vi "AGE_Machine_Interface_v6.vi"() -> ()   [LabVIEW 2016]
uses:
  <vilib>/Analysis/3filter.llb/Filter Passband Type.ctl
  <vilib>/instr/_visa.llb/VISA Configure Serial Port (Instr).vi
  <vilib>/ptbypt/NI_PtbyPt.lvlib
  <vilib>/Analysis/NI_AALBase.lvlib
panel:
  out "input variable":dbl
  out "output variable":dbl
  out "Winds Completed":dbl
  out "Total Number of Winds":dbl
  out "sh_r-new":dbl
  out "winds\ncompleted":i32
  out "Roboteq":refnum<visa-resource-name>
  out "Interface Information:Interface Description 2":string
  out "General Settings:Resource Name 2":string
  out "General Settings:Resource Name":string
  out "Interface Information:Interface Description":string
  out "Uno":refnum<visa-resource-name>
  out "List of card in the Computer 2":string[](array[string])
  out "List of card in the Computer":string[](array[string])
  in  "Start Button":bool
  out "READY":bool
  out "INITIALIZING":bool
  out "NOT READY":bool
  in  "Glue Cart":bool
  in  "Fiber Roll":bool
  in  "Acrylic Tube":bool
  out "sh_r":dbl format="%#_5g"
  out "AGE Fiber Outer Diameter [mm]":dbl format="%#_3g"
  out "AGE Length of Roll Wound [m]":dbl format="%#_3g"
  out "AGE Number of Fiber Layers":dbl format="%#_3g"
  out "AGE Length of Roll Wound [ft]":dbl format="%#_3g"
  out "AGE Fiber Outer Diameter [in]":dbl format="%#_3g"
  in  "AGE Fiber \nSurface Area [m^2]":dbl=1.0
  in  "AGE Effective Width [mm]":dbl=50.0
  in  "AGE Initial \nDiameter [in]":dbl=1.0
  out "Quantity Glue":dbl=23.78296263980416 format="%#_2g"
  in  "Motors Stop":bool
  in  "?":bool
  out "error out 2":errorcluster
  out "Ready 2":bool
  out "Ready":bool
  in  "?":bool
  out "error out":errorcluster
  in  "Calculate\nCalculate Button":bool
  in  "Reset Button":bool
  # "AGE Winding Machine Interface"
  # "Serial Port\nStatus"
  # "Setup Operation"
  # "Stepper\nMotor"
  # "Glue Quantity Per Cartridge"
  # "[mL]"
  # "Glue &Wind Motor"
  # "ENTER THE VALUES AND THEN PRESS CALCULATE"
  # "Calculation Outputs"
  # "CHECK THE BOXES IF CRITERIA IS MET BEFORE START"
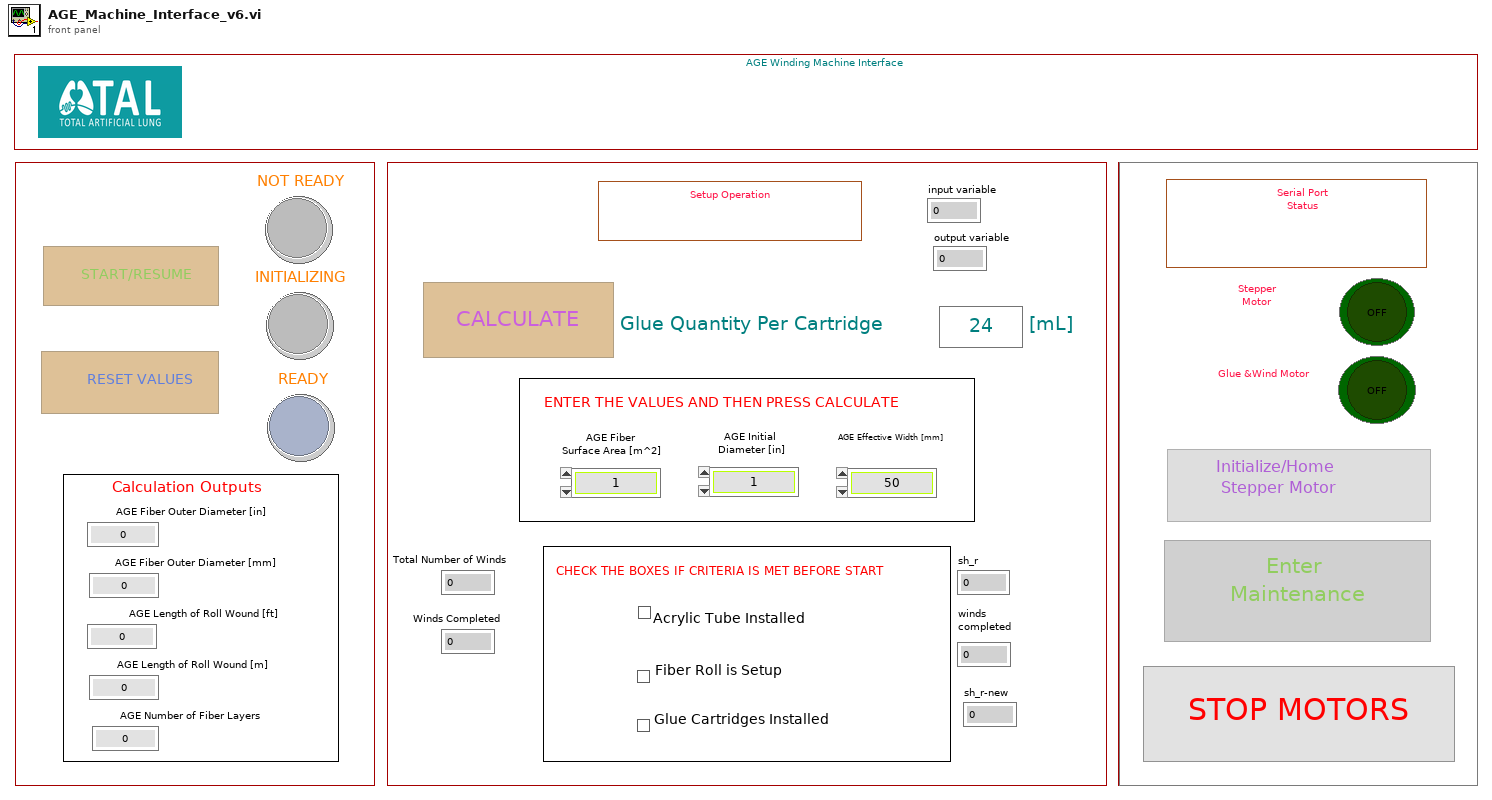
[diagram p1: front panel]
types:
  T1 = cluster{"baud rate":u32, "data bits":u16, "parity":enum16{"None", "Odd", "Even", "Mark", "Space"}, "stop bits":u16, "flow control":u16}
  T2 = typedef "NI_AALBase.lvlib/Filter Passband Type.ctl" = enum32{"Lowpass", "Highpass", "Bandpass", "Bandstop"}
  T3 = enum8{"Enabled", "Disabled", "Disabled and Grayed Out"}
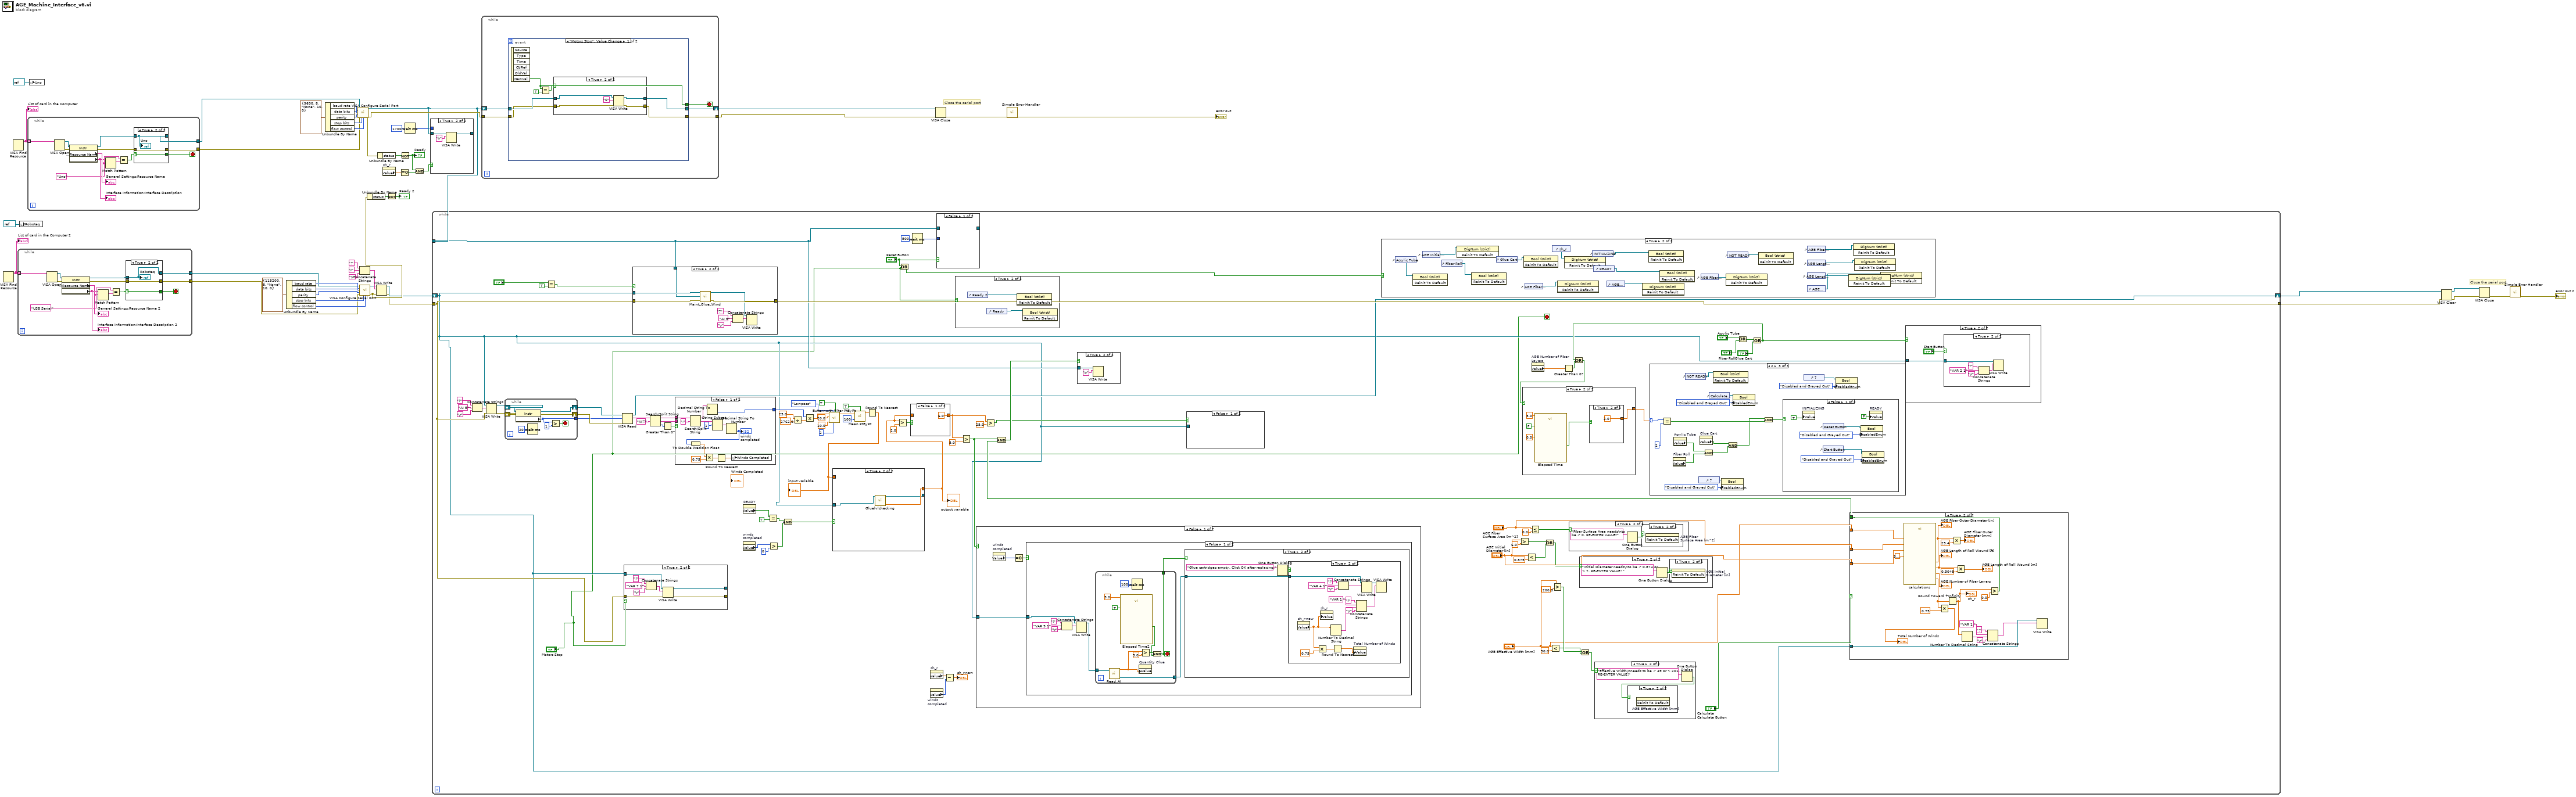
[diagram p0: block diagram]
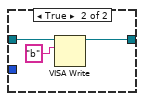
[diagram p5: hidden frame]
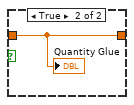
[diagram p7: hidden frame]
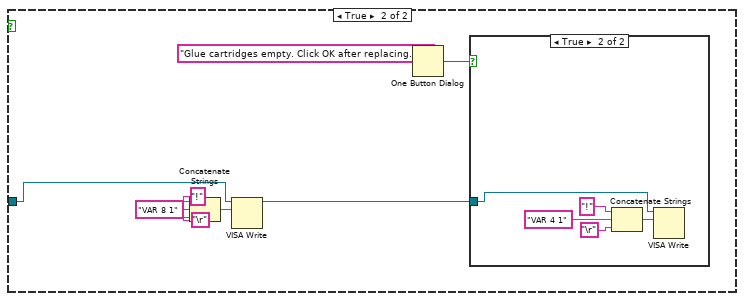
[diagram p10: hidden frame]
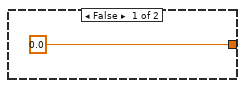
[diagram p14: hidden frame]
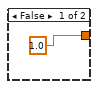
[diagram p15: hidden frame]
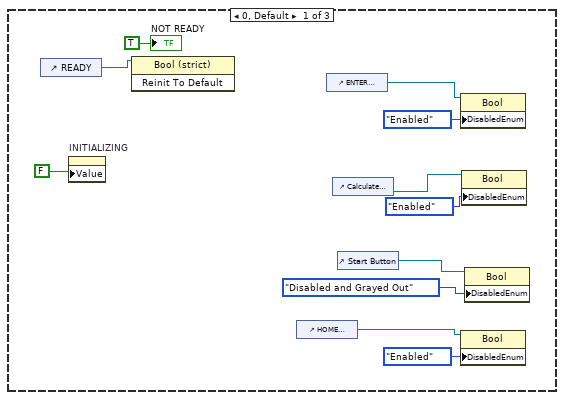
[diagram p16: hidden frame]
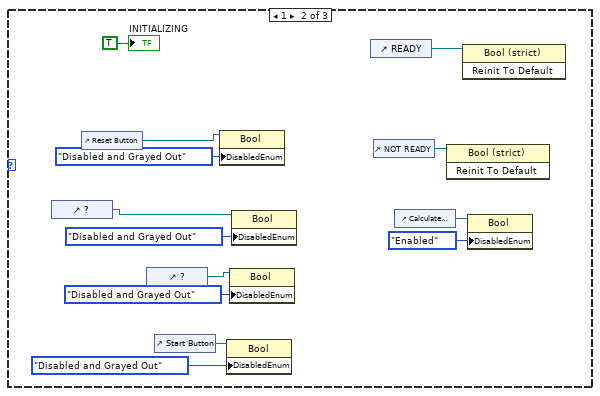
[diagram p17: hidden frame]
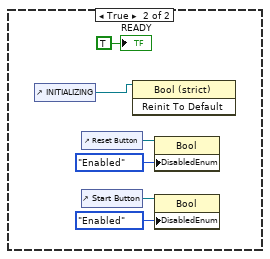
[diagram p18: hidden frame]
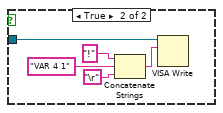
[diagram p19: hidden frame]
diagram:
  # "Close the serial port"
  # "Close the serial port"
  n1 = VISA Find Resource() -> (3:w24:string[])  [unwired: 3 in, 2 out]
  "List of card in the Computer 2" <- w24
  n2 = VISA Find Resource() -> (3:w26:string[])  [unwired: 3 in, 2 out]
  "List of card in the Computer" <- w26
  n3 = while {
    tunnel: w24 -> [w60] mode=indexing
    tunnel: [w54] -> w22
    tunnel: [w52] -> w1
    stop <- w50 stop-if-true
    w55 = "USB Serial" ("Keyword for Roboteq")
    n4 = VISA Open(VISA resource name=w60) -> (VISA resource name=w61:refnum<visa-resource-name>, error out=w62:errorcluster)  [unwired: 4 in]
    n5 = property class="Instr"(reference=w61, error in=w62) -> (reference out=w51:refnum<visa-resource-name>, error out=w53:errorcluster, "General Settings:Resource Name"=→"General Settings:Resource Name 2":string, "Interface Information:Interface Description"=w57:string)
    "Interface Information:Interface Description 2" <- w57
    n6 = Match Pattern(string=w57, regular expression=w55) -> (match substring=w58:string)  [unwired: 1 in, 3 out]
    n7 = Equal?(x=w55, y=w58) -> (x = y?=w59:bool)
    n8 = case shown="True" w59 {
      selector: w59 -> [_ w63]
      tunnel: w51 -> [_ w64]
      tunnel: [_ w65] -> w54
      tunnel: w53 -> [_ w65]
      tunnel: [_ w64] -> w52
      tunnel: [_ w63] -> w50
      frame False {
      }
      frame True {
        "Roboteq" <- w64
      }
    }
  }
  n9 = local write "Roboteq"(refnum<visa-resource-name> refnum ("Roboteq")) -> ()
  n10 = while {
    tunnel: w26 -> [w75] mode=indexing
    tunnel: [w70] -> w21
    tunnel: [w68] -> w9
    stop <- w66 stop-if-true
    w72 = "Uno" ("Keyword for Uno")
    n11 = VISA Open(VISA resource name=w75) -> (VISA resource name=w77:refnum<visa-resource-name>, error out=w78:errorcluster)  [unwired: 4 in]
    n12 = property class="Instr"(reference=w77, error in=w78) -> (reference out=w67:refnum<visa-resource-name>, error out=w69:errorcluster, "General Settings:Resource Name"=→"General Settings:Resource Name":string, "Interface Information:Interface Description"=w71:string)
    "Interface Information:Interface Description" <- w71
    n13 = Match Pattern(string=w71, regular expression=w72) -> (match substring=w73:string)  [unwired: 1 in, 3 out]
    n14 = Equal?(x=w72, y=w73) -> (x = y?=w74:bool)
    n15 = case shown="True" w74 {
      selector: w74 -> [_ w80]
      tunnel: w67 -> [_ w79]
      tunnel: [_ w81] -> w70
      tunnel: w69 -> [_ w81]
      tunnel: [_ w79] -> w68
      tunnel: [_ w80] -> w66
      frame False {
      }
      frame True {
        "Uno" <- w79
      }
    }
  }
  n16 = local write "Uno"(refnum<visa-resource-name> refnum ("Uno")) -> ()
  n17 = Unbundle By Name(T1 {"baud rate"=115200, "data bits"=8, "parity"=enum."None", "stop bits"=10, "flow control"=0} ("Serial Settings")) -> ("baud rate"=w38:u32, "data bits"=w37:u16, "parity"=w36:enum16{"None", "Odd", "Even", "Mark", "Space"}, "stop bits"=w35:u16, "flow control"=w34:u16)
  n18 = Unbundle By Name(T1 {"baud rate"=9600, "data bits"=8, "parity"=enum."None", "stop bits"=10, "flow control"=0} ("Serial Settings")) -> ("baud rate"=w43:u32, "data bits"=w44:u16, "parity"=w45:enum16{"None", "Odd", "Even", "Mark", "Space"}, "stop bits"=w46:u16, "flow control"=w47:u16)
  n19 = call-poly "VISA Configure Serial Port"("VISA resource name"=w9, "baud rate (9600)"=w43, "data bits (8)"=w44, "parity (0:none)"=w45, "error in (no error)"=w21, "stop bits (10: 1 bit)"=w46, "flow control (0:none)"=w47) -> ("VISA resource name out"=w4:refnum<visa-resource-name>, "error out"=w10:errorcluster)  [unwired: 7 in]
  n20 = Concatenate Strings("!" ("string to write 2"), "r" ("string"), "\r") -> (w29:string)
  n21 = call-poly "VISA Configure Serial Port"("VISA resource name"=w1, "baud rate (9600)"=w38, "data bits (8)"=w37, "parity (0:none)"=w36, "error in (no error)"=w22, "stop bits (10: 1 bit)"=w35, "flow control (0:none)"=w34) -> ("VISA resource name out"=w20:refnum<visa-resource-name>, "error out"=w19:errorcluster)  [unwired: 7 in]
  n22 = Unbundle By Name(w19) -> ("status"=w40:bool)
  n23 = VISA Write(VISA resource name=w20, write buffer=w29, error in (no error)=w19) -> (VISA resource name out=w14:refnum<visa-resource-name>, error out=w13:errorcluster)  [unwired: 1 out]
  n24 = Unbundle By Name(w10) -> ("status"=w41:bool)
  n25 = property on="sh_r" class="DigNum (strict)"() -> ("Value"=w8:dbl)  [unwired: 2 in, 2 out]
  n26 = Not(x=w40) -> (.not. x?=→"Ready 2":bool)
  n27 = Equal To 0?(x=w8) -> (x = 0?=w7:bool)
  n28 = Not(x=w41) -> (.not. x?=w6:bool)
  "Ready" <- w6
  n29 = Wait (ms)(milliseconds to wait=u32 1700) -> (millisecond timer value=w2:u32)
  n30 = And(x=w6, y=w7) -> (x .and. y?=w5:bool)
  n31 = case shown="True" w5 {
    tunnel: w4 -> [_ w83]
    tunnel: [_ w82] -> _
    tunnel: w2 -> [_ _]
    frame False {
    }
    frame True {
      n32 = VISA Write(VISA resource name=w83, write buffer="b") -> (VISA resource name out=w82:refnum<visa-resource-name>)  [unwired: 1 in, 2 out]
    }
  }
  n33 = while {
    tunnel: [w172] -> w16
    tunnel: w13 -> [w171]
    shift-right: [w114] -> w18
    shift-left: w14 -> [w86]
    tunnel: w4 -> [w89]
    stop <- "Motors Stop" stop-if-true
    n34 = Concatenate Strings("?" ("string to write 2"), "AI 5" ("string"), "\r") -> (w147:string)
    n35 = VISA Write(VISA resource name=w86, write buffer=w147, error in (no error)=w171) -> (VISA resource name out=w149:refnum<visa-resource-name>, error out=w151:errorcluster)  [unwired: 1 out]
    n36 = while {
      shift-right: [w330] -> w152
      shift-left: w151 -> [w329]
      shift-right: [w327] -> w148
      shift-left: w149 -> [w328]
      tunnel: [w324] -> w124
      stop <- w325 stop-if-true
      n37 = property class="Instr"(reference=w328, error in=w329) -> (reference out=w327:refnum<visa-resource-name>, error out=w330:errorcluster, "Serial Settings:Number of Bytes at Serial Port"=w324:u32)
      n38 = Wait (ms)(milliseconds to wait=u32 20) -> ()  [unwired: 1 out]
      n39 = Greater?(x=w324, y=u32 1) -> (0:w325:bool)
    }
    n40 = Equal?(x="?", y=TRUE) -> (x = y?=w168:bool)
    n41 = VISA Read(VISA resource name=w148, byte count=w124, error in (no error)=w152) -> (VISA resource name out=w114:refnum<visa-resource-name>, read buffer=w138:string)  [unwired: 2 out]
    n42 = case shown="True" "Motors Stop" {
      tunnel: w86 -> [_ w380]
      tunnel: w171 -> [_ w379]
      tunnel: [_ w378] -> _
      tunnel: [_ w377] -> _
      frame False {
      }
      frame True {
        n43 = Concatenate Strings("!" ("string to write 2"), "VAR 7 1" ("string"), "\r") -> (w373:string)
        n44 = VISA Write(VISA resource name=w380, write buffer=w373, error in (no error)=w379) -> (VISA resource name out=w377:refnum<visa-resource-name>, error out=w378:errorcluster)  [unwired: 1 out]
      }
    }
    n45 = case shown="True" w168 {
      tunnel: w86 -> [_ w371]
      tunnel: w171 -> [_ w370]
      tunnel: [_ w372] -> w172
      tunnel: w89 -> [_ w369]
      frame False {
      }
      frame True {
        n46 = call "Maint_Glue_Wind.vi"("VISA Refnum in"=w371, "VISA Refnum in 2"=w369, "error in (no error)"=w370) -> ("VISA Refnum out"=w364:refnum<visa-resource-name>, "error out"=w372:errorcluster)  [unwired: 10 in, 1 out]
        n47 = Concatenate Strings("?" ("string to write 2"), "AI 5" ("string"), "\r") -> (w367:string)
        n48 = VISA Write(VISA resource name=w364, write buffer=w367) -> ()  [unwired: 1 in, 3 out]
      }
    }
    n49 = Search/Split String(string=w138, search string/char (-)="AI=") -> (substring before match=w139:string, match + rest of string=w142:string, offset of match=w141:i32)  [unwired: 1 in]
    n50 = Greater Than 0?(x=w141) -> (x > 0?=w140:bool)
    n51 = case shown="False" w140 {
      tunnel: [w315 w319] -> w162
      tunnel: w142 -> [_ w321]
      tunnel: w139 -> [w317 _]
      frame False {
        n52 = Search/Split String(string=w317, search string/char (-)="-") -> (substring before match=w316:string, match + rest of string=w314:string)  [unwired: 1 in, 1 out]
        n53 = Decimal String To Number(string=w316) -> (number=w315:i32)  [unwired: 2 in, 1 out]
        n54 = String Subset(string=w314, offset (0)=1) -> (substring=w312:string)  [unwired: 1 in]
        n55 = Decimal String To Number(string=w312) -> (number=w311:i32)  [unwired: 2 in, 1 out]
        "winds\ncompleted" <- w311
        n56 = To Double Precision Float(number=w311) -> (double precision float=w310:dbl)
        n57 = Multiply(x=w310, y=0.75) -> (x*y=w308:dbl)
        n58 = Round To Nearest(number=w308) -> (nearest integer value=w307:dbl)
        n59 = local write "Winds Completed"(w307) -> ()
      }
      frame True {
        n60 = String Subset(string=w321, offset (0)=3) -> (substring=w320:string)  [unwired: 1 in]
        n61 = Decimal String To Number(string=w320) -> (number=w319:i32)  [unwired: 2 in, 1 out]
      }
    }
    n62 = property on="winds\ncompleted" class="DigNum (strict)"() -> ("Value"=w94:i32)  [unwired: 2 in, 2 out]
    n63 = property on="READY" class="Bool (strict)"() -> ("Value"=w101:bool)  [unwired: 2 in, 2 out]
    n64 = Equal?(x=w101, y=TRUE) -> (x = y?=w95:bool)
    n65 = Greater?(x=w94, y=0) -> (0:w93:bool)
    n66 = And(x=w95, y=w93) -> (x .and. y?=w91:bool)
    n67 = Divide(x=25.0, y=2762.0) -> (x/y=w161:dbl)
    n68 = Multiply(x=w162, y=w161) -> (x*y=w153:dbl)
    n69 = call <vilib>:"Butterworth Filter PtByPt.vi"("initialize"=TRUE, "order"=2, "filter type"=Filter_Passband_Type."Lowpass", "low cutoff freq: fl"=10.0, "sampling freq: fs"=20.0, "x"=w153) -> ("Filtered x"=w112:dbl)  [unwired: 3 in, 1 out]
    n70 = call <vilib>:"Mean PtByPt.vi"("x"=w112, "sample length"=100, "initialize"=TRUE) -> ("mean"=w111:dbl)  [unwired: 1 in, 1 out]
    n71 = Round To Nearest(number=w111) -> (nearest integer value=w100:dbl)
    "input variable" <- w100
    n72 = case shown="True" w91 {
      tunnel: w100 -> [w176 _]
      tunnel: [w176 w179] -> w97
      tunnel: [_ w178] -> _
      tunnel: w86 -> [_ w177]
      frame False {
      }
      frame True {
        n73 = call "Gluelvlchecking.vi"("VISA resource name"=w177) -> ("QG"=w179:dbl, "VISA resource name out"=w178:refnum<visa-resource-name>)  [unwired: 9 in]
      }
    }
    "output variable" <- w97
    n74 = Greater?(x=w97, y=2.0) -> (0:w98:bool)
    n75 = Or(x="Reset Button", y="Motors Stop") -> (x .or. y?=w106:bool)
    n76 = case shown="False" w98 {
      tunnel: w97 -> [_ w181]
      tunnel: [6.0 w181] -> w96
      frame False {
      }
      frame True {
        "Quantity Glue" <- w181
      }
    }
    n77 = Wait (ms)(milliseconds to wait=u32 500) -> (millisecond timer value=w87:u32)
    n78 = property on="sh_r" class="DigNum (strict)"() -> ("Value"=w119:dbl)  [unwired: 2 in, 2 out]
    n79 = property on="winds\ncompleted" class="DigNum (strict)"() -> ("Value"=w118:i32)  [unwired: 2 in, 2 out]
    n80 = case shown="False" "Reset Button" {
      tunnel: w89 -> [_ w174]
      tunnel: [_ w173] -> _
      tunnel: w87 -> [_ _]
      frame False {
      }
      frame True {
        n81 = VISA Write(VISA resource name=w174, write buffer="b") -> (VISA resource name out=w173:refnum<visa-resource-name>)  [unwired: 1 in, 2 out]
      }
    }
    n82 = Subtract(x=w119, y=w118) -> (x-y=→"sh_r-new":dbl)
    n83 = case shown="True" "Motors Stop" {
      frame False {
      }
      frame True {
        n84 = control-ref of="Ready 2"() -> (w234:refnum<vi>)
        n85 = control-ref of="Ready"() -> (w235:refnum<vi>)
        n86 = invoke class="Bool (strict)" method="Reinit To Default"(reference=w234) -> ()  [unwired: 2 in, 3 out]
        n87 = invoke class="Bool (strict)" method="Reinit To Default"(reference=w235) -> ()  [unwired: 2 in, 3 out]
      }
    }
    n88 = Greater?(x=w96, y=5.0) -> (0:w103:bool)
    n89 = case shown="False" w103 {
      tunnel: w86 -> [w183 _]
      frame False {
        n90 = property on="winds\ncompleted" class="DigNum (strict)"() -> ("Value"=w182:i32)  [unwired: 2 in, 2 out]
        n91 = Equal To 0?(x=w182) -> (x = 0?=w184:bool)
        n92 = case shown="False" w184 {
          tunnel: w183 -> [w192 w224]
          frame False {
            n93 = Concatenate Strings("!" ("string to write 2"), "VAR 9 1" ("string"), "\r") -> (w189:string)
            n94 = VISA Write(VISA resource name=w192, write buffer=w189) -> (VISA resource name out=w187:refnum<visa-resource-name>)  [unwired: 1 in, 2 out]
            n95 = while {
              tunnel: w187 -> [w213]
              tunnel: [w212] -> w186
              tunnel: [w215] -> w185
              stop <- w215 stop-if-true
              n96 = call "Read_AI.vi"("VISA resource name"=w213) -> ("VISA resource name out"=w212:refnum<visa-resource-name>, "Numeric"=w211:dbl)  [unwired: 9 in]
              n97 = call "Elapsed Time2"("Time Target (s)"=9.0, "Auto Reset"=TRUE) -> ("Time has Elapsed"=w216:bool)  [unwired: 10 in, 7 out]
              n98 = Wait (ms)(milliseconds to wait=u32 100 ("millisecond timer value")) -> ()  [unwired: 1 out]
              n99 = property on="Quantity Glue" class="DigNum (strict)"("Value"=w211) -> ()  [unwired: 2 in, 2 out]
              n100 = Greater?(x=w211, y=5.0) -> (0:w218:bool)
              n101 = And(x=w218, y=w216) -> (x .and. y?=w215:bool)
            }
            n102 = case shown="True" w185 {
              tunnel: w186 -> [_ w193]
              frame False {
              }
              frame True {
                n103 = One Button Dialog(message="Glue cartridges empty. Click OK after replacing.") -> (true=w194:bool)  [unwired: 1 in]
                n104 = case shown="True" w194 {
                  tunnel: w193 -> [_ w206]
                  frame False {
                  }
                  frame True {
                    n105 = property on="sh_r-new" class="DigNum (strict)"() -> ("Value"=w199:dbl)  [unwired: 2 in, 2 out]
                    n106 = Multiply(x=w199, y=0.75) -> (x*y=w197:dbl)
                    n107 = property on="sh_r" class="DigNum (strict)"("Value"=w199) -> ()  [unwired: 2 in, 2 out]
                    n108 = Number To Decimal String(number=w199) -> (decimal integer string=w201:string)  [unwired: 1 in]
                    n109 = Round To Nearest(number=w197) -> (nearest integer value=w196:dbl)
                    n110 = Concatenate Strings("!" ("string to write 2"), "VAR 4 1" ("string"), "\r") -> (w209:string)
                    n111 = property on="Total Number of Winds" class="DigNum (strict)"("Value"=w196) -> ()  [unwired: 2 in, 2 out]
                    n112 = Concatenate Strings("!" ("string to write 2"), "VAR 1 " ("string"), w201, "\r") -> (w203:string)
                    n113 = VISA Write(VISA resource name=w206, write buffer=w209) -> (VISA resource name out=w200:refnum<visa-resource-name>)  [unwired: 1 in, 2 out]
                    n114 = VISA Write(VISA resource name=w200, write buffer=w203) -> ()  [unwired: 1 in, 3 out]
                  }
                }
              }
            }
          }
          frame True {
            n115 = Concatenate Strings("!" ("string to write 2"), "VAR 8 1" ("string"), "\r") -> (w226:string)
            n116 = VISA Write(VISA resource name=w224, write buffer=w226) -> (VISA resource name out=w221:refnum<visa-resource-name>)  [unwired: 1 in, 2 out]
            n117 = One Button Dialog(message="Glue cartridges empty. Click OK after replacing.") -> (true=w222:bool)  [unwired: 1 in]
            n118 = case shown="True" w222 {
              tunnel: w221 -> [_ w229]
              frame False {
              }
              frame True {
                n119 = Concatenate Strings("!" ("string to write 2"), "VAR 4 1" ("string"), "\r") -> (w232:string)
                n120 = VISA Write(VISA resource name=w229, write buffer=w232) -> ()  [unwired: 1 in, 3 out]
              }
            }
          }
        }
      }
      frame True {
      }
    }
    n121 = Greater?(x=w96, y=25.0) -> (0:w113:bool)
    n122 = case shown="False" w113 {
      tunnel: w86 -> [_ w296]
      frame False {
      }
      frame True {
        n123 = Concatenate Strings("!" ("string to write 2"), "VAR 4 1" ("string"), "\r") -> (w298:string)
        n124 = VISA Write(VISA resource name=w296, write buffer=w298) -> ()  [unwired: 1 in, 3 out]
      }
    }
    n125 = case shown="True" w106 {
      frame False {
      }
      frame True {
        n126 = control-ref of="Acrylic Tube"() -> (w395:refnum<vi>)
        n127 = invoke class="Bool (strict)" method="Reinit To Default"(reference=w395) -> ()  [unwired: 2 in, 3 out]
        n128 = control-ref of="AGE Initial \nDiameter [in]"() -> (w387:refnum<vi>)
        n129 = control-ref of="Fiber Roll"() -> (w394:refnum<vi>)
        n130 = invoke class="DigNum (strict)" method="Reinit To Default"(reference=w387) -> ()  [unwired: 2 in, 3 out]
        n131 = invoke class="Bool (strict)" method="Reinit To Default"(reference=w394) -> ()  [unwired: 2 in, 3 out]
        n132 = control-ref of="Glue Cart"() -> (w393:refnum<vi>)
        n133 = invoke class="Bool (strict)" method="Reinit To Default"(reference=w393) -> ()  [unwired: 2 in, 3 out]
        n134 = control-ref of="AGE Fiber \nSurface Area [m^2]"() -> (w389:refnum<vi>)
        n135 = control-ref of="sh_r"() -> (w386:refnum<vi>)
        n136 = invoke class="DigNum (strict)" method="Reinit To Default"(reference=w389) -> ()  [unwired: 2 in, 3 out]
        n137 = invoke class="DigNum (strict)" method="Reinit To Default"(reference=w386) -> ()  [unwired: 2 in, 3 out]
        n138 = control-ref of="INITIALIZING"() -> (w390:refnum<vi>)
        n139 = control-ref of="READY"() -> (w391:refnum<vi>)
        n140 = control-ref of="AGE Effective Width [mm]"() -> (w388:refnum<vi>)
        n141 = invoke class="DigNum (strict)" method="Reinit To Default"(reference=w388) -> ()  [unwired: 2 in, 3 out]
        n142 = invoke class="Bool (strict)" method="Reinit To Default"(reference=w390) -> ()  [unwired: 2 in, 3 out]
        n143 = invoke class="Bool (strict)" method="Reinit To Default"(reference=w391) -> ()  [unwired: 2 in, 3 out]
        n144 = control-ref of="AGE Fiber Outer Diameter [in]"() -> (w385:refnum<vi>)
        n145 = invoke class="DigNum (strict)" method="Reinit To Default"(reference=w385) -> ()  [unwired: 2 in, 3 out]
        n146 = control-ref of="NOT READY"() -> (w392:refnum<vi>)
        n147 = invoke class="Bool (strict)" method="Reinit To Default"(reference=w392) -> ()  [unwired: 2 in, 3 out]
        n148 = control-ref of="AGE Length of Roll Wound [m]"() -> (w382:refnum<vi>)
        n149 = control-ref of="AGE Number of Fiber Layers"() -> (w381:refnum<vi>)
        n150 = control-ref of="AGE Fiber Outer Diameter [mm]"() -> (w384:refnum<vi>)
        n151 = control-ref of="AGE Length of Roll Wound [ft]"() -> (w383:refnum<vi>)
        n152 = invoke class="DigNum (strict)" method="Reinit To Default"(reference=w382) -> ()  [unwired: 2 in, 3 out]
        n153 = invoke class="DigNum (strict)" method="Reinit To Default"(reference=w384) -> ()  [unwired: 2 in, 3 out]
        n154 = invoke class="DigNum (strict)" method="Reinit To Default"(reference=w383) -> ()  [unwired: 2 in, 3 out]
        n155 = invoke class="DigNum (strict)" method="Reinit To Default"(reference=w381) -> ()  [unwired: 2 in, 3 out]
      }
    }
    n156 = Greater?(x="AGE Initial \nDiameter [in]", y=6.0) -> (0:w129:bool)
    n157 = Less?(x="AGE Initial \nDiameter [in]", y=0.875) -> (x < y?=w127:bool)
    n158 = Less Or Equal?(x="AGE Fiber \nSurface Area [m^2]", y=0.0) -> (x <= y?=w122:bool)
    n159 = property on="AGE Number of Fiber Layers" class="DigNum (strict)"() -> ("Value"=w116:dbl)  [unwired: 2 in, 2 out]
    n160 = Or(x=w129, y=w127) -> (x .or. y?=w121:bool)
    n161 = Less?(x="AGE Effective Width [mm]", y=50.0) -> (x < y?=w135:bool)
    n162 = Greater?(x="AGE Effective Width [mm]", y=200.0) -> (0:w137:bool)
    n163 = Greater Than 0?(x=w116) -> (x > 0?=w117:bool)
    n164 = case shown="True" w122 {
      frame False {
      }
      frame True {
        n165 = One Button Dialog(message="Fiber Surface Area needs\nto be > 0. RE-ENTER VALUE!") -> (true=w303:bool)  [unwired: 1 in]
        n166 = case shown="True" w303 {
          frame False {
          }
          frame True {
            n167 = invoke on="AGE Fiber \nSurface Area [m^2]" class="DigNum (strict)" method="Reinit To Default"() -> ()  [unwired: 3 in, 3 out]
          }
        }
      }
    }
    n168 = case shown="True" w121 {
      frame False {
      }
      frame True {
        n169 = One Button Dialog(message="Initial Diameter needs\nto be > 0.874 or < 7. RE-ENTER VALUE! ") -> (true=w301:bool)  [unwired: 1 in]
        n170 = case shown="True" w301 {
          frame False {
          }
          frame True {
            n171 = invoke on="AGE Initial \nDiameter [in]" class="DigNum (strict)" method="Reinit To Default"() -> ()  [unwired: 3 in, 3 out]
          }
        }
      }
    }
    n172 = Or(x=w137, y=w135) -> (x .or. y?=w132:bool)
    n173 = case shown="True" w132 {
      frame False {
      }
      frame True {
        n174 = One Button Dialog(message="Effective Width\nneeds to be > 49 or < 201. RE-ENTER VALUE!") -> (true=w305:bool)  [unwired: 1 in]
        n175 = case shown="True" w305 {
          frame False {
          }
          frame True {
            n176 = invoke on="AGE Effective Width [mm]" class="DigNum (strict)" method="Reinit To Default"() -> ()  [unwired: 3 in, 3 out]
          }
        }
      }
    }
    n177 = Or(x="Acrylic Tube", y="Fiber Roll") -> (x .or. y?=w165:bool)
    n178 = Or(x=w165, y="Glue Cart") -> (x .or. y?=w105:bool)
    n179 = Or(x=w105, y=w117) -> (x .or. y?=w108:bool)
    n180 = case shown="True" w108 {
      tunnel: [0.0 w241] -> w107
      frame False {
      }
      frame True {
        n181 = call "Elapsed Time"("Time Target (s)"=5.0, "Auto Reset"=FALSE, "Set Start Time (s)"=0.0) -> ("Time has Elapsed"=w237:bool)  [unwired: 9 in, 7 out]
        n182 = case shown="True" w237 {
          tunnel: [1.0 2.0] -> w241
          frame False {
          }
          frame True {
          }
        }
      }
    }
    n183 = case shown="2" w107 {
      selector: w107 -> [_ _ w276]
      frame 0, Default {
        n184 = control-ref of="READY"() -> (w247:refnum<vi>)
        n185 = property on="INITIALIZING" class="Bool (strict)"("Value"=FALSE) -> ()  [unwired: 2 in, 2 out]
        n186 = invoke class="Bool (strict)" method="Reinit To Default"(reference=w247) -> ()  [unwired: 2 in, 3 out]
        n187 = control-ref of="HOME STEPPER MOTOR"() -> (w244:refnum<vi>)
        n188 = control-ref of="ENTER MAINTENANCE"() -> (w245:refnum<vi>)
        n189 = control-ref of="Calculate\nCalculate Button"() -> (w250:refnum<vi>)
        n190 = control-ref of="Start Button"() -> (w253:refnum<vi>)
        n191 = property class="Bool"(reference=w245, "DisabledEnum"=T3."Enabled" ("Disabled")) -> ()  [unwired: 1 in, 2 out]
        n192 = property class="Bool"(reference=w244, "DisabledEnum"=T3."Enabled" ("Disabled")) -> ()  [unwired: 1 in, 2 out]
        n193 = property class="Bool"(reference=w250, "DisabledEnum"=T3."Enabled" ("Disabled")) -> ()  [unwired: 1 in, 2 out]
        n194 = property class="Bool"(reference=w253, "DisabledEnum"=T3."Disabled and Grayed Out" ("Disabled")) -> ()  [unwired: 1 in, 2 out]
        "NOT READY" <- TRUE
      }
      frame 1 {
        n195 = control-ref of="?"() -> (w263:refnum<vi>)
        n196 = control-ref of="Reset Button"() -> (w257:refnum<vi>)
        n197 = control-ref of="?"() -> (w259:refnum<vi>)
        n198 = control-ref of="Start Button"() -> (w265:refnum<vi>)
        n199 = property class="Bool"(reference=w257, "DisabledEnum"=T3."Disabled and Grayed Out" ("Disabled")) -> ()  [unwired: 1 in, 2 out]
        n200 = property class="Bool"(reference=w265, "DisabledEnum"=T3."Disabled and Grayed Out" ("Disabled")) -> ()  [unwired: 1 in, 2 out]
        n201 = property class="Bool"(reference=w259, "DisabledEnum"=T3."Disabled and Grayed Out" ("Disabled")) -> ()  [unwired: 1 in, 2 out]
        n202 = property class="Bool"(reference=w263, "DisabledEnum"=T3."Disabled and Grayed Out" ("Disabled")) -> ()  [unwired: 1 in, 2 out]
        n203 = control-ref of="READY"() -> (w255:refnum<vi>)
        n204 = control-ref of="NOT READY"() -> (w266:refnum<vi>)
        n205 = control-ref of="Calculate\nCalculate Button"() -> (w261:refnum<vi>)
        n206 = invoke class="Bool (strict)" method="Reinit To Default"(reference=w266) -> ()  [unwired: 2 in, 3 out]
        n207 = invoke class="Bool (strict)" method="Reinit To Default"(reference=w255) -> ()  [unwired: 2 in, 3 out]
        n208 = property class="Bool"(reference=w261, "DisabledEnum"=T3."Enabled" ("Disabled")) -> ()  [unwired: 1 in, 2 out]
        "INITIALIZING" <- TRUE
      }
      frame 2 {
        n209 = Equal?(x=w276, y=2) -> (x = y?=w274:bool)
        n210 = property on="Fiber Roll" class="Bool (strict)"() -> ("Value"=w271:bool)  [unwired: 2 in, 2 out]
        n211 = property on="Acrylic Tube" class="Bool (strict)"() -> ("Value"=w272:bool)  [unwired: 2 in, 2 out]
        n212 = control-ref of="NOT READY"() -> (w283:refnum<vi>)
        n213 = control-ref of="?"() -> (w278:refnum<vi>)
        n214 = property on="Glue Cart" class="Bool (strict)"() -> ("Value"=w269:bool)  [unwired: 2 in, 2 out]
        n215 = And(x=w272, y=w271) -> (x .and. y?=w270:bool)
        n216 = control-ref of="Calculate\nCalculate Button"() -> (w282:refnum<vi>)
        n217 = invoke class="Bool (strict)" method="Reinit To Default"(reference=w283) -> ()  [unwired: 2 in, 3 out]
        n218 = property class="Bool"(reference=w278, "DisabledEnum"=T3."Disabled and Grayed Out" ("Disabled")) -> ()  [unwired: 1 in, 2 out]
        n219 = And(x=w269, y=w270) -> (x .and. y?=w268:bool)
        n220 = property class="Bool"(reference=w282, "DisabledEnum"=T3."Disabled and Grayed Out" ("Disabled")) -> ()  [unwired: 1 in, 2 out]
        n221 = And(x=w268, y=w274) -> (x .and. y?=w273:bool)
        n222 = case shown="False" w273 {
          frame False {
            n223 = property on="INITIALIZING" class="Bool (strict)"("Value"=TRUE) -> ()  [unwired: 2 in, 2 out]
            n224 = control-ref of="Start Button"() -> (w286:refnum<vi>)
            n225 = control-ref of="Reset Button"() -> (w287:refnum<vi>)
            n226 = property class="Bool"(reference=w287, "DisabledEnum"=T3."Disabled and Grayed Out" ("Disabled")) -> ()  [unwired: 1 in, 2 out]
            n227 = property class="Bool"(reference=w286, "DisabledEnum"=T3."Disabled and Grayed Out" ("Disabled")) -> ()  [unwired: 1 in, 2 out]
            n228 = property on="READY" class="Bool (strict)"("Value"=FALSE) -> ()  [unwired: 2 in, 2 out]
          }
          frame True {
            n229 = control-ref of="INITIALIZING"() -> (w291:refnum<vi>)
            n230 = control-ref of="Reset Button"() -> (w292:refnum<vi>)
            n231 = control-ref of="Start Button"() -> (w295:refnum<vi>)
            n232 = invoke class="Bool (strict)" method="Reinit To Default"(reference=w291) -> ()  [unwired: 2 in, 3 out]
            n233 = property class="Bool"(reference=w292, "DisabledEnum"=T3."Enabled" ("Disabled")) -> ()  [unwired: 1 in, 2 out]
            n234 = property class="Bool"(reference=w295, "DisabledEnum"=T3."Enabled" ("Disabled")) -> ()  [unwired: 1 in, 2 out]
            "READY" <- TRUE ("READY")
          }
        }
        n235 = control-ref of="?"() -> (w280:refnum<vi>)
        n236 = property class="Bool"(reference=w280, "DisabledEnum"=T3."Disabled and Grayed Out" ("Disabled")) -> ()  [unwired: 1 in, 2 out]
      }
    }
    n237 = case shown="True" "Calculate\nCalculate Button" {
      tunnel: w86 -> [_ w353]
      tunnel: [_ w338] -> w143
      tunnel: "AGE Effective Width [mm]" -> [_ w336]
      tunnel: "AGE Fiber \nSurface Area [m^2]" -> [_ w335]
      tunnel: "AGE Initial \nDiameter [in]" -> [_ w334]
      frame False {
      }
      frame True {
        n238 = call "calculations.vi"("pi"=3.141592653589793, "AGE Initial \nDiameter [in]"=w334, "AGE Effective Width [mm]"=w336, "AGE Fiber \nSurface Area [m^2]"=w335) -> ("l_w"=w343:dbl, "n"=→"AGE Number of Fiber Layers":dbl, "age_od"=w346:dbl, "sh_r"=w333:dbl)  [unwired: 4 in]
        "AGE Fiber Outer Diameter [in]" <- w346
        "AGE Length of Roll Wound [ft]" <- w343
        n239 = Multiply(x=w333, y=0.75) -> (x*y=→"Total Number of Winds":dbl)
        n240 = Round Toward +Infinity(x=w333) -> (ceil(x): smallest int >= x=w337:dbl)
        "sh_r" <- w337
        n241 = Multiply(x=w346, y=25.4) -> (x*y=→"AGE Fiber Outer Diameter [mm]":dbl)
        n242 = Multiply(x=w343, y=0.3048) -> (x*y=→"AGE Length of Roll Wound [m]":dbl)
        n243 = Number To Decimal String(number=w337) -> (decimal integer string=w340:string)  [unwired: 1 in]
        n244 = Concatenate Strings("!" ("string to write 2"), "VAR 1 " ("string"), w340, "\r") -> (w350:string)
        n245 = Greater?(x=w337, y=0.0) -> (0:w338:bool)
        n246 = VISA Write(VISA resource name=w353, write buffer=w350) -> ()  [unwired: 1 in, 3 out]
      }
    }
    n247 = And(x=w103, y=w143) -> (x .and. y?=w163:bool)
    n248 = case shown="True" w163 {
      tunnel: w89 -> [_ w363]
      frame False {
      }
      frame True {
        n249 = VISA Write(VISA resource name=w363, write buffer="p") -> ()  [unwired: 1 in, 3 out]
      }
    }
    n250 = case shown="True" w105 {
      tunnel: w86 -> [_ w356]
      frame False {
        n251 = control-ref of="READY"() -> (w354:refnum<vi>)
        n252 = invoke class="Bool (strict)" method="Reinit To Default"(reference=w354) -> ()  [unwired: 2 in, 3 out]
      }
      frame True {
        n253 = case shown="True" "Start Button" {
          tunnel: w356 -> [_ w357]
          frame False {
          }
          frame True {
            n254 = Concatenate Strings("!" ("string to write 2"), "VAR 2 1" ("string"), "\r") -> (w359:string)
            n255 = VISA Write(VISA resource name=w357, write buffer=w359) -> ()  [unwired: 1 in, 3 out]
          }
        }
      }
    }
  }
  n256 = while {
    tunnel: w10 -> [w397]
    tunnel: [w398] -> w11
    shift-right: [w399] -> w12
    shift-left: w4 -> [w396]
    stop <- w400 stop-if-true
    n257 = event shown="[0] \"Motors Stop\": Value Change" {
      selector: _ -> [_ _]
      dyn-events: _ -> [_ _]
      timeout: _ -> [_ _]
      tunnel: w396 -> [w404 w416]
      tunnel: w397 -> [w403 w417]
      tunnel: [w406 _] -> w400
      tunnel: [w402 w415] -> w399
      tunnel: [w401 w414] -> w398
      event "Motors Stop": Value Change {
        n258 = event-data() -> ("NewVal"=w406:bool)  [unwired: 1 in, 5 out]
        n259 = Equal?(x=w406, y=TRUE) -> (x = y?=w407:bool)
        n260 = case shown="True" w407 {
          tunnel: w404 -> [_ w408]
          tunnel: w403 -> [_ w409]
          tunnel: [_ w411] -> w402
          tunnel: [_ w410] -> w401
          frame False {
          }
          frame True {
            n261 = VISA Write(VISA resource name=w408, write buffer="S", error in (no error)=w409) -> (VISA resource name out=w411:refnum<visa-resource-name>, error out=w410:errorcluster)  [unwired: 1 out]
          }
        }
      }
      event Value Change {
        n262 = event-data() -> ()  [unwired: 1 in, 6 out]
        n263 = VISA Write(VISA resource name=w416, write buffer="i", error in (no error)=w417) -> (VISA resource name out=w415:refnum<visa-resource-name>, error out=w414:errorcluster)  [unwired: 1 out]
      }
    }
  }
  n264 = VISA Close(VISA resource name=w12, error in (no error)=w11) -> (error out=w49:errorcluster)
  n265 = call <vilib>:"Simple Error Handler.vi"("error in (no error)"=w49) -> ("error out"=→"error out":errorcluster)  [unwired: 1 in, 7 out]
  n266 = VISA Clear(VISA resource name=w18, error in (no error)=w16) -> (VISA resource name out=w17:refnum<visa-resource-name>, error out=w15:errorcluster)
  n267 = VISA Close(VISA resource name=w17, error in (no error)=w15) -> (error out=w33:errorcluster)
  n268 = call <vilib>:"Simple Error Handler.vi"("error in (no error)"=w33) -> ("error out"=→"error out 2":errorcluster)  [unwired: 1 in, 7 out]
